vi "RunTimeMissing Dialog.vi"(5 "error in":errorcluster) -> (19 "error out":errorcluster)   [LabVIEW 2018, in "LcWebView.lvclass"]
uses:
  LcWebView.lvclass
  <vilib>/Platform/browser.llb/Open URL in Default Browser (string).vi
panel:
  in  "View Button":bool
  in  "Close":bool
  in  "Exit":bool
  in  "Download":bool
  out "Link":string
  # "Webview2 Run-Time engine missing"
  # "This application required the Webview2 Run-Time engine,\nwhich couldn't be found.\n\nPlease install this and restart the application.\n\nDownload it from here:"
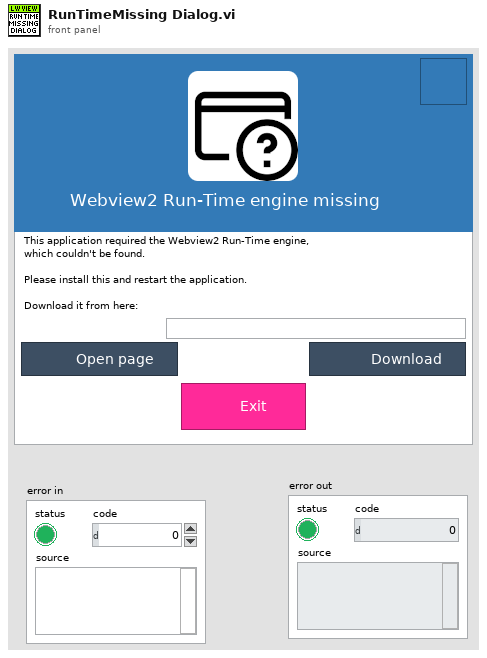
[diagram p1: front panel]
types:
  T1 = typedef "LVRectTypeDef.ctl" = cluster{"Left":i16, "Top":i16, "Right":i16, "Bottom":i16}
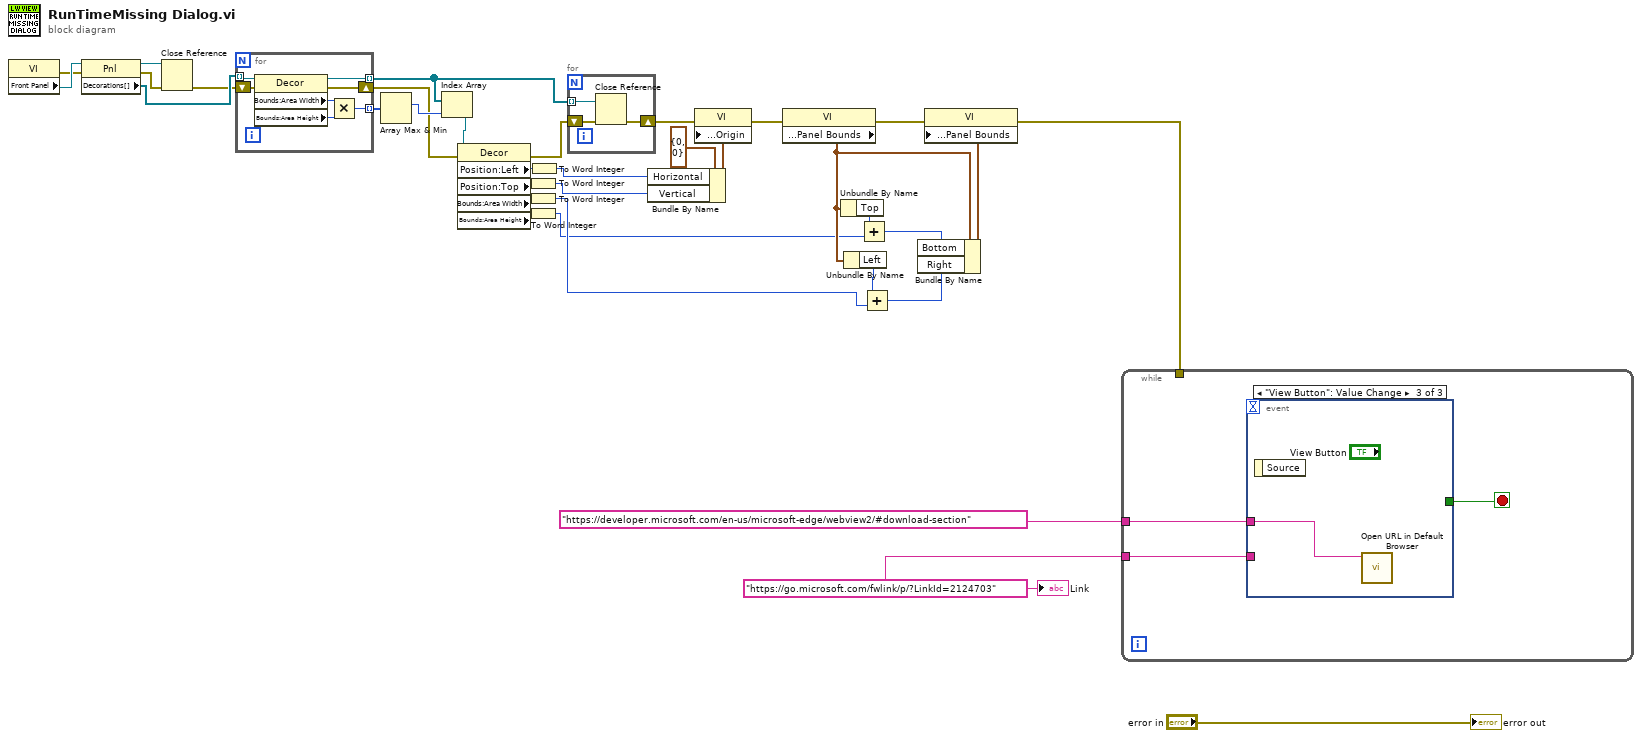
[diagram p0: block diagram]
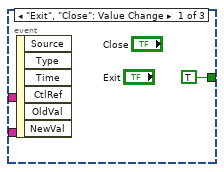
[diagram p2: hidden frame]
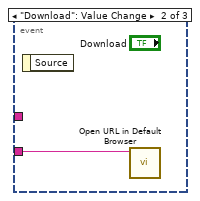
[diagram p3: hidden frame]
diagram:
  w35 = "https://go.microsoft.com/fwlink/p/?LinkId=2124703" ("Link")
  n1 = property on="Property Node" class="VI"() -> (error out=w29:errorcluster, "Front Panel"=w31:refnum<vi>)  [unwired: 2 in, 1 out]
  n2 = property on="Property Node" class="Pnl"(reference=w31, error in=w29) -> (reference out=w28:refnum<vi>, error out=w30:errorcluster, "Decorations[]"=w33:refnum<vi>[])
  n3 = Close Reference(reference=w28, error in (no error)=w30) -> (error out=w32:errorcluster)
  n4 = for {
    tunnel: w33 -> [w42] mode=indexing
    tunnel: [w39] -> w16 mode=indexing
    shift-right: [w37] -> w12
    shift-left: w32 -> [w38]
    tunnel: [w36] -> w14 mode=indexing
    n5 = property class="Decor"(reference=w42, error in=w38) -> (reference out=w36:refnum<vi>, error out=w37:errorcluster, "Bounds:Area Width"=w41:u32, "Bounds:Area Height"=w40:u32)
    n6 = Multiply(x=w41, y=w40) -> (x*y=w39:u32)
  }
  n7 = Array Max & Min(array=w16) -> (max index (indices)=w15:i32)  [unwired: 3 out]
  n8 = Index Array(array=w14, index=w15) -> (element=w13:refnum<vi>)
  n9 = property class="Decor"(reference=w13, error in=w12) -> (error out=w11:errorcluster, "Position:Left"=w19:i32, "Position:Top"=w20:i32, "Bounds:Area Width"=w25:u32, "Bounds:Area Height"=w23:u32)  [unwired: 1 out]
  n10 = To Word Integer(number=w20) -> (16bit integer=w4:i16)
  n11 = To Word Integer(number=w25) -> (16bit integer=w7:i16)
  n12 = To Word Integer(number=w23) -> (16bit integer=w6:i16)
  n13 = To Word Integer(number=w19) -> (16bit integer=w5:i16)
  n14 = for {
    tunnel: w14 -> [w45] mode=indexing
    shift-right: [w43] -> w10
    shift-left: w11 -> [w44]
    n15 = Close Reference(reference=w45, error in (no error)=w44) -> (error out=w43:errorcluster)
  }
  n16 = Bundle By Name(cluster=cluster{"Horizontal":i16, "Vertical":i16} {"Horizontal"=0, "Vertical"=0} ("Front Panel Window:Origin"), "Horizontal"=w5, "Vertical"=w4) -> (w17:cluster{"Horizontal":i16, "Vertical":i16})
  n17 = property on="Property Node" class="VI"(error in=w10, "Front Panel Window:Origin"=w17) -> (error out=w9:errorcluster)  [unwired: 1 in, 1 out]
  n18 = property on="Property Node" class="VI"(error in=w9) -> (error out=w8:errorcluster, "Front Panel Window:Panel Bounds"=w21:T1)  [unwired: 1 in, 1 out]
  n19 = Unbundle By Name(w21) -> ("Top"=w22:i16)
  n20 = Unbundle By Name(w21) -> ("Left"=w24:i16)
  n21 = Add(x=w22, y=w6) -> (x+y=w3:i16)
  n22 = Add(x=w24, y=w7) -> (x+y=w2:i16)
  n23 = Bundle By Name(cluster=w21, "Bottom"=w3, "Right"=w2) -> (w26:T1)
  n24 = property on="Property Node" class="VI"(error in=w8, "Front Panel Window:Panel Bounds"=w26) -> (error out=w27:errorcluster)  [unwired: 1 in, 1 out]
  n25 = while {
    tunnel: w35 -> [w47]
    tunnel: w27 -> [_]
    tunnel: "https://developer.microsoft.com/en-us/microsoft-edge/webview2/#download-section" ("Link") -> [w46]
    stop <- w48 stop-if-true
    n26 = event shown="[2] \"View Button\": Value Change" {
      selector: _ -> [_ _ _]
      dyn-events: _ -> [_ _ _]
      timeout: _ -> [_ _ _]
      tunnel: [TRUE _ _] -> w48
      tunnel: w47 -> [_ w50 _]
      tunnel: w46 -> [_ _ w51]
      event "Exit", "Close": Value Change {
        n27 = event-data() -> ()  [unwired: 1 in, 6 out]
      }
      event "Download": Value Change {
        n28 = event-data() -> ()  [unwired: 1 in, 1 out]
        n29 = call-poly <vilib>:"Open URL in Default Browser.vi"("URL"=w50) -> ()  [unwired: 5 in, 2 out]
      }
      event "View Button": Value Change {
        n30 = event-data() -> ()  [unwired: 1 in, 1 out]
        n31 = call-poly <vilib>:"Open URL in Default Browser.vi"("URL"=w51) -> ()  [unwired: 5 in, 2 out]
      }
    }
  }
  "Link" <- w35
  "error out" <- "error in"
